vi "activateESC.vi"(2 "error in (no error)":errorcluster) -> (0 "error out":errorcluster, 1 "PWM Ref Out":T1)   [LabVIEW 2021]
uses:
  <vilib>/myRIO/Instrument Drivers/Onboard IO/PWM/typedefs/PWM Reference.ctl
  <vilib>/myRIO/Common/Instrument Driver Framework/Utilities/typedefs/myRIO Generic Hardware Reference.ctl
  <vilib>/myRIO/Common/Instrument Driver Framework/Utilities/typedefs/Hardware Version Enum.ctl
  <vilib>/myRIO/Common/Instrument Driver Framework/Utilities/typedefs/myRIO v1.0 Reference.ctl
  <vilib>/myRIO/Common/Instrument Driver Framework/Utilities/typedefs/Generic FPGA Reference.ctl
  <vilib>/myRIO/Common/Instrument Driver Framework/myRIO v1.0/PWM/typedefs/PWM Channels Enum.ctl
  <vilib>/myRIO/Instrument Drivers/Onboard IO/PWM/typedefs/PWM Configuration.ctl
  <vilib>/Utility/error.llb/Error Cluster From Error Code.vi
  <vilib>/myRIO/Common/Instrument Driver Framework/myRIO v1.0/PWM/vis/myRIO v1.0 Write PWM.vi
  <vilib>/myRIO/Instrument Drivers/Onboard IO/PWM/PWM.lvlib
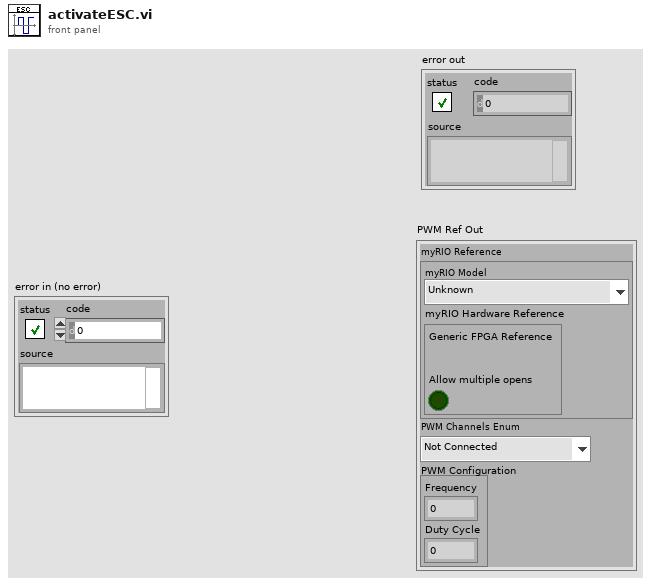
[diagram p1: front panel]
types:
  T1 = typedef "PWM.lvlib/PWM Reference.ctl" = cluster{"myRIO Reference":T2, "PWM Channels Enum":T6, "PWM Configuration":T7}
  T2 = typedef "myRIO Generic Hardware Reference.ctl" = cluster{"myRIO Model":T3, "myRIO Hardware Reference":T4}
  T3 = typedef "Hardware Version Enum.ctl" = enum16{"Unknown", "myRIO-1900", "myRIO-1950", "roboRIO", "NI ELVIS RIO CM", "ELVIS III"}
  T4 = typedef "myRIO v1.0 Reference.ctl" = cluster{"Generic FPGA Reference":T5, "Allow multiple opens":bool}
  T5 = typedef "Generic FPGA Reference.ctl" = refnum<k20>
  T6 = typedef "PWM Channels Enum.ctl" = enum16{"Not Connected", "C/PWM0", "C/PWM1", "A/PWM0", "A/PWM1", "A/PWM2", "A/PWM3", "A/PWM4", "A/PWM5", "A/PWM6", "A/PWM7", "A/PWM8", "A/PWM9", "A/PWM10", "A/PWM11", "A/PWM12", "A/PWM13", "A/PWM14", "A/PWM15", "A/PWM16", "A/PWM17", "A/PWM18", "A/PWM19", "B/PWM0", "B/PWM1", "B/PWM2", "B/PWM3", "B/PWM4", "B/PWM5", "B/PWM6", "B/PWM7", "B/PWM8", "B/PWM9", "B/PWM10", "B/PWM11", "B/PWM12", "B/PWM13", "B/PWM14", "B/PWM15", "B/PWM16", "B/PWM17", "B/PWM18", "B/PWM19", "PWM/PWM0", "PWM/PWM1", "PWM/PWM2", "PWM/PWM3", "PWM/PWM4", "PWM/PWM5", "PWM/PWM6", "PWM/PWM7", "PWM/PWM8", "PWM/PWM9"}
  T7 = typedef "PWM.lvlib/PWM Configuration.ctl" = cluster{"Frequency":dbl, "Duty Cycle":dbl}
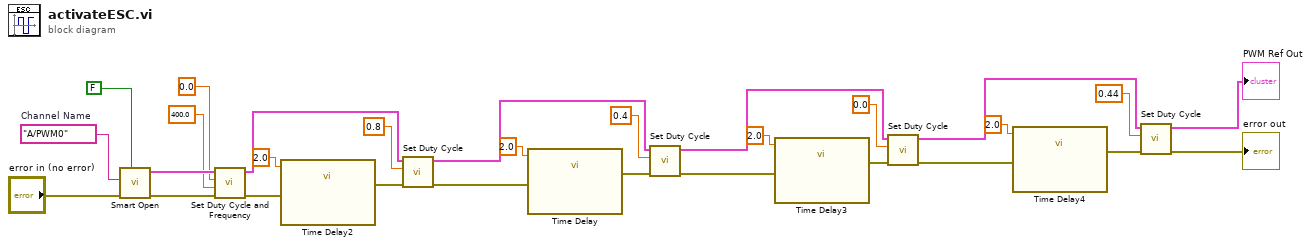
[diagram p0: block diagram]
diagram:
  w29 = tag "A/PWM0"  # Channel Name
  n1 = call <vilib>:"Smart Open.vi"("Allow multiple opens?"=FALSE, "error in (no error)"="error in (no error)", "Channel Name"=w29) -> ("error out"=w27:errorcluster, "PWM Ref Out"=w28:T1)  [unwired: 7 in]
  n2 = call <vilib>:"Set Duty Cycle and Frequency.vi"("error in (no error)"=w27, "Frequency [Hz]"=400.0, "Duty Cycle"=0.0, "PWM Ref In"=w28) -> ("error out"=w23:errorcluster, "PWM Ref Out"=w17:T1)  [unwired: 5 in]
  n3 = call "Time Delay2"("error in (no error)"=w23, "Delay Time (s)"=2.0) -> ("error out"=w18:errorcluster)  [unwired: 9 in]
  n4 = call <vilib>:"Set Duty Cycle.vi"("error in (no error)"=w18, "Duty Cycle"=0.8, "PWM Ref In"=w17) -> ("error out"=w21:errorcluster, "PWM Ref Out"=w14:T1)  [unwired: 6 in]
  n5 = call "Time Delay"("error in (no error)"=w21, "Delay Time (s)"=2.0) -> ("error out"=w16:errorcluster)  [unwired: 9 in]
  n6 = call <vilib>:"Set Duty Cycle.vi"("error in (no error)"=w16, "Duty Cycle"=0.4, "PWM Ref In"=w14) -> ("error out"=w13:errorcluster, "PWM Ref Out"=w10:T1)  [unwired: 6 in]
  n7 = call "Time Delay3"("error in (no error)"=w13, "Delay Time (s)"=2.0) -> ("error out"=w11:errorcluster)  [unwired: 9 in]
  n8 = call <vilib>:"Set Duty Cycle.vi"("error in (no error)"=w11, "Duty Cycle"=0.0, "PWM Ref In"=w10) -> ("error out"=w7:errorcluster, "PWM Ref Out"=w5:T1)  [unwired: 6 in]
  n9 = call "Time Delay4"("error in (no error)"=w7, "Delay Time (s)"=2.0) -> ("error out"=w6:errorcluster)  [unwired: 9 in]
  n10 = call <vilib>:"Set Duty Cycle.vi"("error in (no error)"=w6, "Duty Cycle"=0.44, "PWM Ref In"=w5) -> ("error out"=→"error out":errorcluster, "PWM Ref Out"=→"PWM Ref Out":T1)  [unwired: 6 in]
